vi "Actor Core.vi"(8 "error in":errorcluster, 11 "Measure Object in":refnum<class "VI Server Recorder.lvclass">) -> (0 "error out":errorcluster, 3 "Actor out":refnum<class "Actor.lvclass">)   [LabVIEW 2019, in "VI Server Recorder.lvclass"]
doc: "(<B>Filename</B>: Actor Framework.lvlib:Actor.lvclass:Actor Core.vi)\n\nReceives messages to the actor, reacts to them, and initiates any error handling that may shut the actor down.\n\nDescendant classes may override this VI to append parallel tasks for the actor to complete while it handles messages. Overrides use the Call Parent Method node."
uses:
  VI Server Recorder.lvclass
  <vilib>/ActorFramework/Actor/Actor.lvclass
  VI Server Configuration.ctl
  Worker/Worker.lvclass
panel:
  in  "Configuration":T1={"Machine name (\"\":  open local reference)"="localhost", "Port number (3363)"=3380, "Control names"=["X"], "VI  name"="Test.vi"}
  out "Name":string
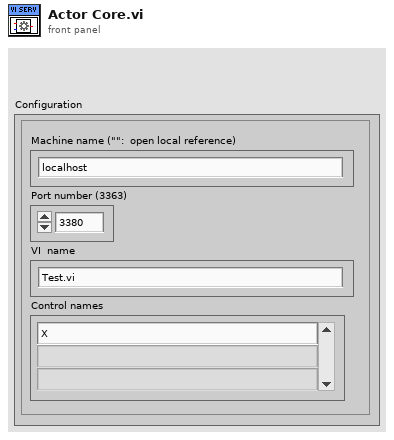
[diagram p1: front panel]
types:
  T1 = typedef "VI Server Configuration.ctl" = cluster{"Machine name (\"\":  open local reference)":string, "Port number (3363)":u16, "Control names":string[], "VI  name":string}
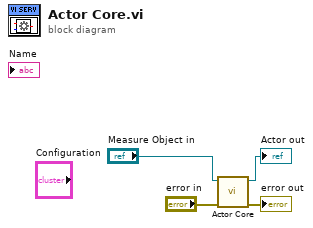
[diagram p0: block diagram]
diagram:
  n1 = call-parent "Actor Core.vi"("error in"="error in", "Measure Object in"="Measure Object in") -> ("error out"=→"error out":errorcluster, "Actor out"=→"Actor out":refnum<class "Actor.lvclass">)  [unwired: 8 in]
